vi "_Convert to DAC Value.vi"(6 "Neg Polarity (F)":bool, 8 "Offset":dbl, 9 "Slop":dbl, 10 "Number":dbl, 11 "Channel":i32=1) -> (1 "DAC Value":i32)   [LabVIEW 2015]
uses:
  _Global Configuration.vi
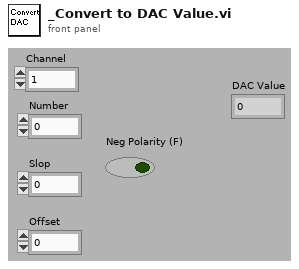
[diagram p1: front panel]
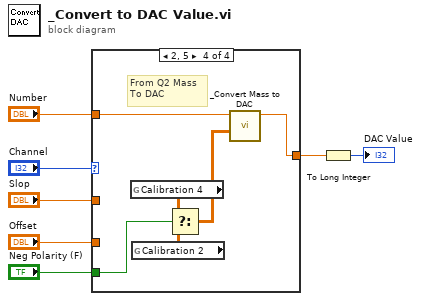
[diagram p0: block diagram]
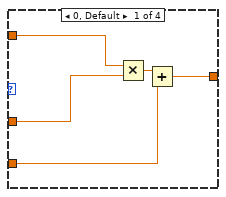
[diagram p2: hidden frame]
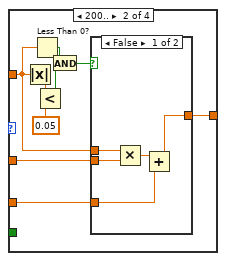
[diagram p3: hidden frame]
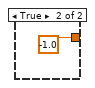
[diagram p4: hidden frame]
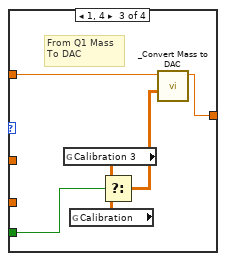
[diagram p5: hidden frame]
diagram:
  n1 = case shown="2, 5" "Channel" {
    tunnel: "Number" -> [w12 w14 w33 w39]
    tunnel: [w11 w16 w32 w38] -> w5
    tunnel: "Slop" -> [w9 w15 _ _]
    tunnel: "Offset" -> [w8 w13 _ _]
    tunnel: "Neg Polarity (F)" -> [_ _ w29 w37]
    frame 0, Default {
      n2 = Multiply(x=w12, y=w9) -> (x*y=w10:dbl)
      n3 = Add(x=w10, y=w8) -> (x+y=w11:dbl)
    }
    frame 200.. {
      n4 = Absolute Value(x=w14) -> (abs(x)=w20:dbl)
      n5 = Less Than 0?(x=w14) -> (x < 0?=w18:bool)
      n6 = Less?(x=w20, y=0.05) -> (x < y?=w17:bool)
      n7 = And(x=w18, y=w17) -> (x .and. y?=w19:bool)
      n8 = case shown="False" w19 {
        tunnel: [w22 -1.0 ("y")] -> w16
        tunnel: w15 -> [w25 _]
        tunnel: w14 -> [w24 _]
        tunnel: w13 -> [w23 _]
        frame False {
          n9 = Multiply(x=w24, y=w25) -> (x*y=w26:dbl)
          n10 = Add(x=w26, y=w23) -> (x+y=w22:dbl)
        }
        frame True {
        }
      }
    }
    frame 1, 4 {
      # "From Q1 Mass\nTo DAC"
      n11 = global read "_Global Configuration.vi" "Calibration 3"() -> (w31:dbl[][])
      n12 = global read "_Global Configuration.vi" "Calibration"() -> (w30:dbl[][])
      n13 = Select(t=w31, s=w29, f=w30) -> (s? t:f=w28:dbl[][])
      n14 = call "_Convert Mass to DAC.vi"("Calibration Table"=w28, "Mass"=w33) -> ("DAC Value"=w32:dbl)  [unwired: 2 in, 3 out]
    }
    frame 2, 5 {
      # "From Q2 Mass\nTo DAC"
      n15 = global read "_Global Configuration.vi" "Calibration 4"() -> (w36:dbl[][])
      n16 = global read "_Global Configuration.vi" "Calibration 2"() -> (w35:dbl[][])
      n17 = Select(t=w36, s=w37, f=w35) -> (s? t:f=w34:dbl[][])
      n18 = call "_Convert Mass to DAC.vi"("Calibration Table"=w34, "Mass"=w39) -> ("DAC Value"=w38:dbl)  [unwired: 2 in, 3 out]
    }
  }
  n19 = To Long Integer(number=w5) -> (32bit integer=→"DAC Value":i32)
